vi "Add.vi"() -> ()   [LabVIEW 2020]
panel:
  out "return value":dbl
  in  "Numeric 2":dbl
  in  "Numeric":dbl
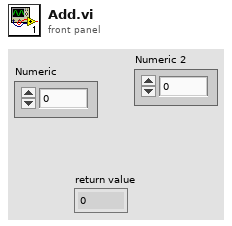
[diagram p1: front panel]
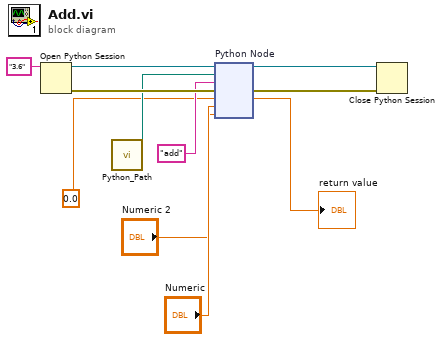
[diagram p0: block diagram]
diagram:
  n1 = Open Python Session(python version="3.6" ("Python version")) -> (session out=w10:refnum<k35>, error out=w9:errorcluster)  [unwired: 2 in]
  n2 = call "Python_Path.vi"() -> ("appended path"=w8:path)  [unwired: 11 in]
  n3 = node "Python Node"(w10, w8, "add" ("function name"), w9, 0.0, "Numeric", "Numeric 2") -> (w2:refnum<k35>, w3:errorcluster, →"return value":dbl)  [unwired: 2 in, 2 out]
  n4 = Close Python Session(session in=w2, error in=w3) -> ()  [unwired: 1 out]
